vi "Day 01 Part 2.vi"(11 "Input":string) -> (3 "Output":i16)   [LabVIEW 2021]
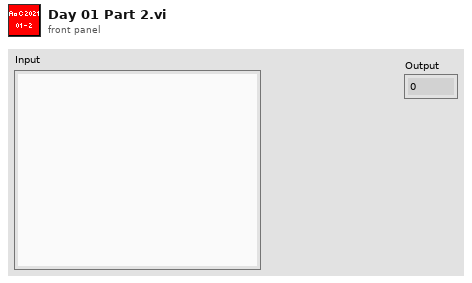
[diagram p1: front panel]
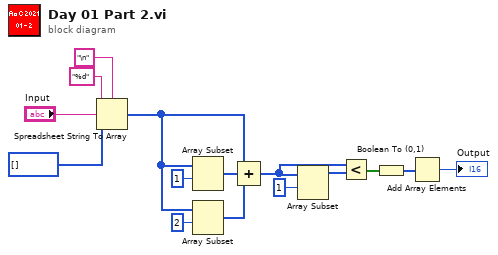
[diagram p0: block diagram]
diagram:
  n1 = Spreadsheet String To Array(delimiter (Tab)="\n", format string="%d", spreadsheet string="Input", array type (2D Dbl)=i32[] []) -> (array=w1:i32[])
  n2 = Array Subset(array=w1, index=1 ("length")) -> (w10:i32[])  [unwired: 1 in]
  n3 = Array Subset(array=w1, index=2 ("length")) -> (w9:i32[])  [unwired: 1 in]
  n4 = Compound Arithmetic op=ADD(w1, w10, w9) -> (w6:i32[])
  n5 = Array Subset(array=w6, index=1 ("length")) -> (w8:i32[])  [unwired: 1 in]
  n6 = Less?(x=w6, y=w8) -> (x < y?=w7:bool[])
  n7 = Boolean To (0,1)(Boolean=w7) -> (0, 1=w14:i16[])
  n8 = Add Array Elements(numeric array=w14) -> (sum=→"Output":i16)
